vi "TDMS Cleanup EMG only.vi"(7 "Accel TDMS File":refnum<k34>, 8 "error in (no error)":errorcluster, 9 "Force TDMS File":refnum<k34>, 10 "TDMS File":path, 11 "Logging in":refnum<class "Logging.lvclass">) -> (0 "error out":errorcluster, 3 "Logging out":refnum<class "Logging.lvclass">)   [LabVIEW 2020, in "Logging.lvlib" / "Logging.lvclass"]
uses:
  Logging.lvclass
  C:/Program Files/National Instruments/LabVIEW 2020/vi.lib/ActorFramework/Actor/Actor.lvclass
  <vilib>/ActorFramework/Actor/Actor.lvclass/Actor.ctl
  <vilib>/ActorFramework/Message Enqueuer/Message Enqueuer.lvclass/Message Enqueuer.ctl
  Logging.lvclass/Logging.ctl
  <vilib>/ActorFramework/Message Enqueuer/Init from Existing Queue.vi
  <vilib>/ActorFramework/Message Enqueuer/Message Enqueuer.lvclass
  <vilib>/ActorFramework/Actor/Actor.lvclass
  Logging Messages/Convert to Excel Msg/Convert to Excel Msg.lvclass
panel:
  out "Numeric":i32
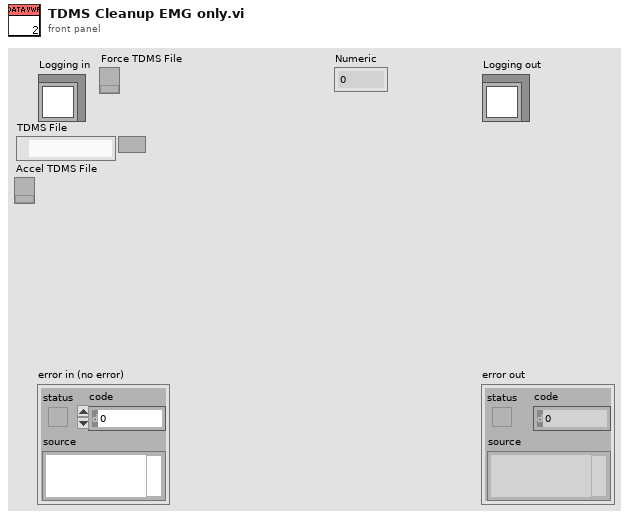
[diagram p1: front panel]
types:
  T1 = enum16{"open", "open or create", "create or replace", "create", "open (read-only)"}
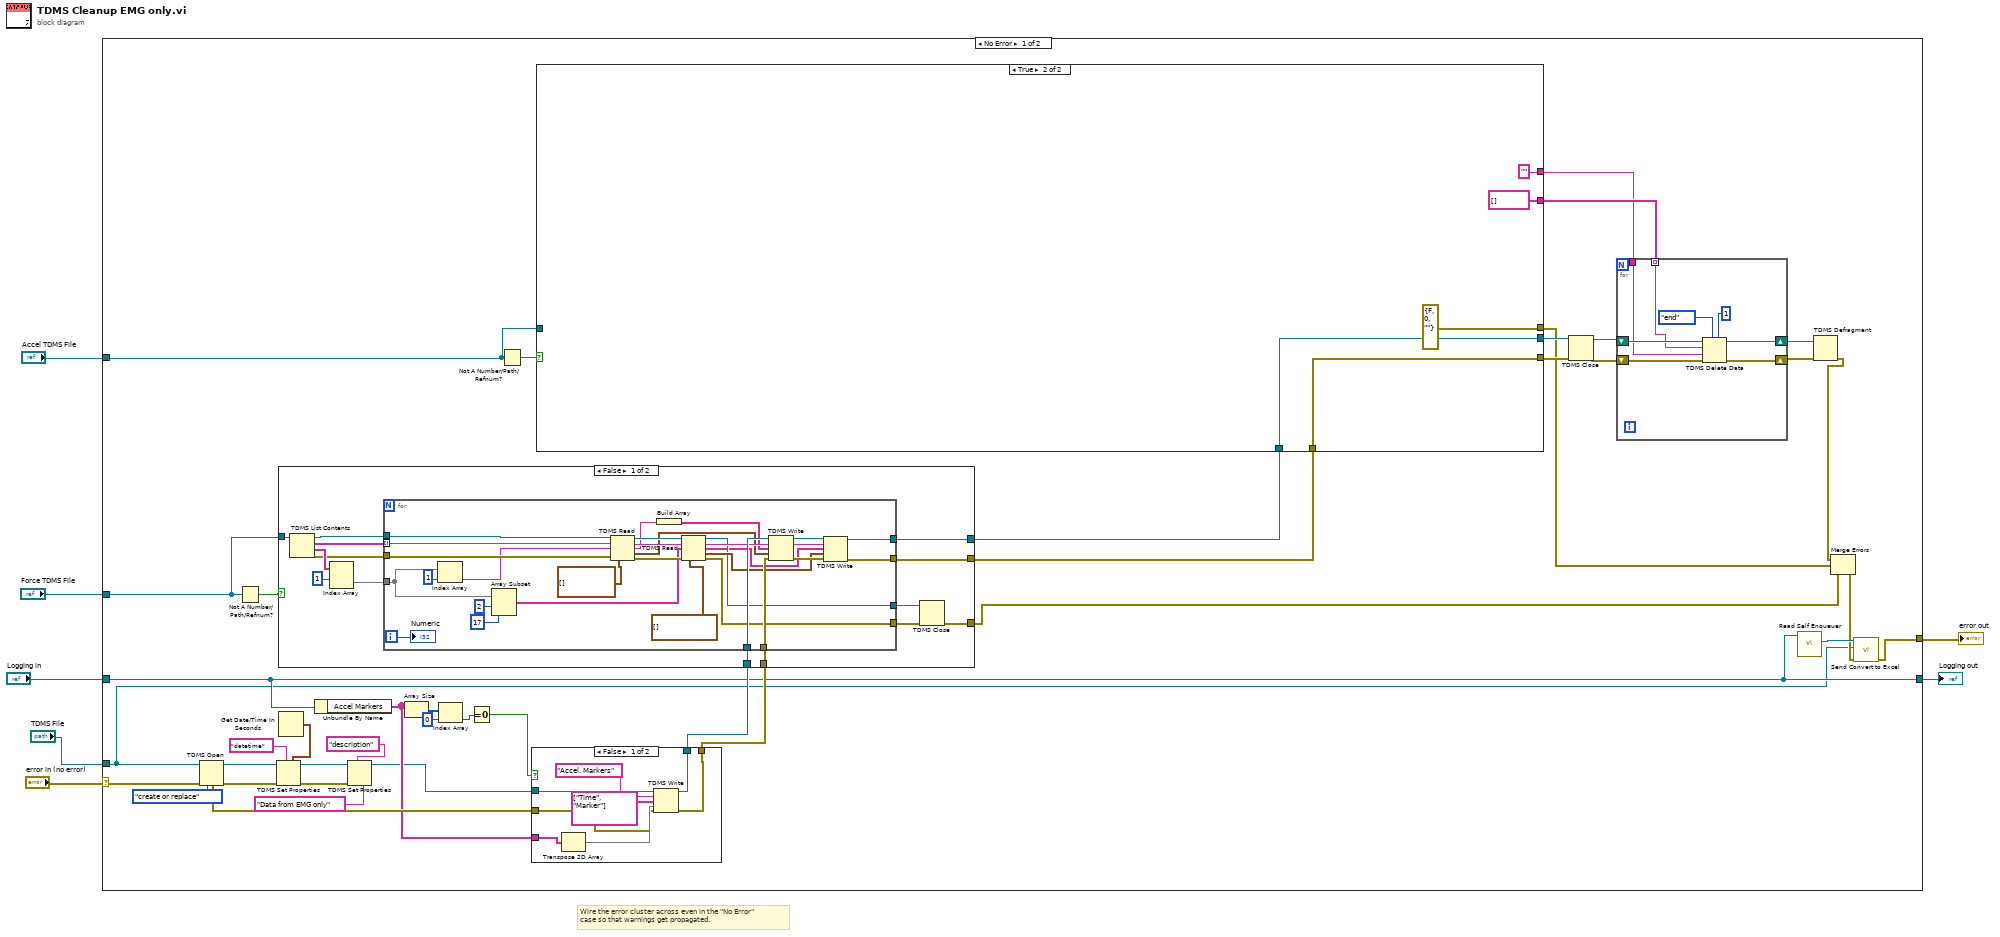
[diagram p0: block diagram]
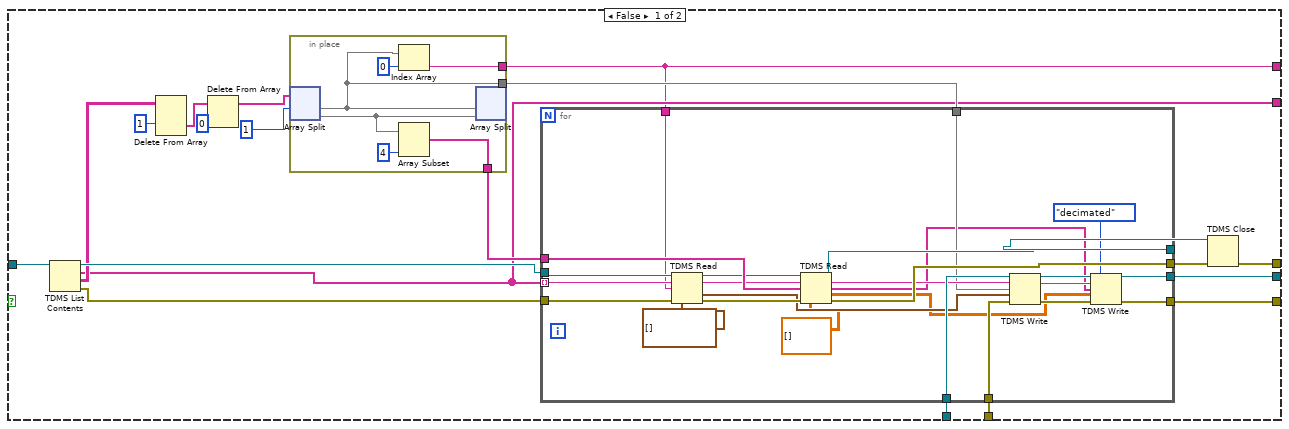
[diagram p2: hidden frame]
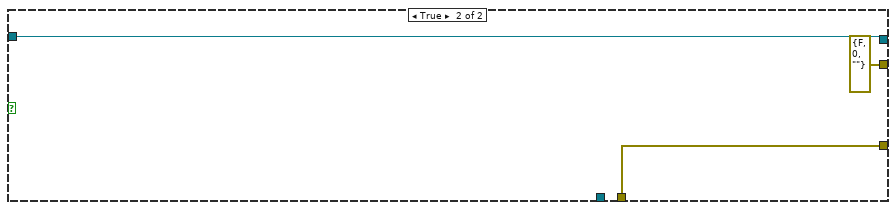
[diagram p3: hidden frame]
diagram:
  # "Wire the error cluster across even in the \"No Error\"\ncase so that warnings get propagated."
  n1 = case shown="No Error" "error in (no error)" {
    selector: "error in (no error)" -> [w41 w171]
    tunnel: [w15 w171] -> w6
    tunnel: [w18 w170] -> w4
    tunnel: "Logging in" -> [w18 w170]
    tunnel: "TDMS File" -> [w14 _]
    tunnel: "Force TDMS File" -> [w31 _]
    tunnel: "Accel TDMS File" -> [w21 _]
    frame No Error {
      n2 = TDMS Open(8:w41, 10:T1."create or replace" ("operation (0:open)"), 11:w14) -> (0:w46:errorcluster, 3:w47:refnum<k34>)  [unwired: 4 in]
      n3 = Not A Number/Path/Refnum?(number/path/refnum=w31) -> (NaN/Path/Refnum?=w32:bool)
      n4 = Get Date/Time In Seconds() -> (seconds since 1Jan1904=w44:timestamp)
      n5 = TDMS Set Properties(5:w44, 7:"datetime", 8:w46, 11:w47) -> (0:w42:errorcluster, 3:w43:refnum<k34>)  [unwired: 2 in, 2 out]
      n6 = Unbundle By Name(w18) -> ("Accel Markers"=w34:string[][])
      n7 = TDMS Set Properties(5:"Data from EMG only" ("property names"), 7:"description" ("property names"), 8:w42, 11:w43) -> (0:w35:errorcluster, 3:w33:refnum<k34>)  [unwired: 2 in, 2 out]
      n8 = Array Size(array=w34) -> (size(s)=w38:i32[])
      n9 = Index Array(array=w38, index=0) -> (element=w36:i32)
      n10 = Equal To 0?(x=w36) -> (x = 0?=w30:bool)
      n11 = Not A Number/Path/Refnum?(number/path/refnum=w21) -> (NaN/Path/Refnum?=w22:bool)
      n12 = case shown="False" w30 {
        tunnel: w33 -> [w167 w169]
        tunnel: w35 -> [w160 w168]
        tunnel: [w164 w169] -> w29
        tunnel: [w163 w168] -> w28
        tunnel: w34 -> [w162 _]
        frame False {
          n13 = Transpose 2D Array(2D array=w162) -> (transposed array=w161:string[][])
          n14 = TDMS Write(0:w167, 5:"Accel. Markers" ("group name in (Untitled)"), 7:string[] ["Time", "Marker"] ("channel name(s) in (Untitled)"), 9:w161, 11:w160) -> (4:w164:refnum<k34>, 15:w163:errorcluster)  [unwired: 1 in, 2 out]
        }
        frame True {
        }
      }
      n15 = case shown="False" w32 {
        tunnel: w31 -> [w126 w159]
        tunnel: w29 -> [w120 _]
        tunnel: w28 -> [w119 w157]
        tunnel: [w115 w157] -> w25
        tunnel: [w114 w159] -> w27
        tunnel: [w113 errorcluster {"status"=FALSE, "code"=0, "source"=""} ("error out")] -> w26
        frame False {
          n16 = TDMS List Contents(7:w126) -> (0:w121:errorcluster, 1:w124:string[][], 2:w123:string[], 3:w118:refnum<k34>)  [unwired: 2 in]
          n17 = Index Array(array=w124, index (row)=1) -> (element=w122:string[])  [unwired: 1 in]
          n18 = for {
            tunnel: w123 -> [w156] mode=indexing
            tunnel: w122 -> [w131]
            tunnel: w121 -> [w152]
            tunnel: w120 -> [w150]
            tunnel: w119 -> [w147]
            tunnel: w118 -> [w146]
            tunnel: [w138] -> w117
            tunnel: [w137] -> w116
            tunnel: [w136] -> w114
            tunnel: [w135] -> w113
            i -> [w133]
            n19 = Index Array(array=w131, index=1) -> (element=w130:string)
            n20 = Array Subset(array=w131, index=2, length=17) -> (w127:string[])
            n21 = TDMS Read(0:w146, 5:w156, 7:w130, 11:w152, 12:timestamp[] []) -> (4:w145:refnum<k34>, 6:w155:string, 8:w142:string, 10:w140:timestamp[], 15:w151:errorcluster)  [unwired: 3 in, 1 out]
            n22 = Build Array(w142) -> (w141:string[])
            n23 = TDMS Read(0:w145, 5:w155, 7:w127, 11:w151, 12:waveform(dbl)[] [] ("data")) -> (4:w138:refnum<k34>, 6:w144:string, 8:w132:string[], 10:w139:waveform(dbl)[], 15:w137:errorcluster)  [unwired: 3 in, 1 out]
            n24 = TDMS Write(0:w150, 5:w144, 7:w141, 9:w140, 11:w147) -> (4:w149:refnum<k34>, 6:w143:string, 15:w148:errorcluster)  [unwired: 1 in, 1 out]
            n25 = TDMS Write(0:w149, 5:w143, 7:w132, 9:w139, 11:w148) -> (4:w136:refnum<k34>, 15:w135:errorcluster)  [unwired: 1 in, 2 out]
            "Numeric" <- w133
          }
          n26 = TDMS Close(8:w116, 11:w117) -> (0:w115:errorcluster)  [unwired: 1 out]
        }
        frame True {
        }
      }
      n27 = case shown="True" w22 {
        tunnel: w21 -> [w76 _]
        tunnel: w27 -> [w74 w112]
        tunnel: [w73 w112] -> w24
        tunnel: w26 -> [w71 w111]
        tunnel: [w69 w111] -> w23
        tunnel: [w68 errorcluster {"status"=FALSE, "code"=0, "source"=""} ("error out")] -> w20
        tunnel: [w58 string[] [] ("group names")] -> w9
        tunnel: [w57 ""] -> w8
        frame False {
          n28 = TDMS List Contents(7:w76) -> (0:w59:errorcluster, 1:w64:string[][], 2:w58:string[], 3:w75:refnum<k34>)  [unwired: 2 in]
          n29 = Delete From Array(array=w64, index (row)=1) -> (deleted portion=w66:string[])  [unwired: 2 in, 1 out]
          n30 = Delete From Array(array=w66, index=0) -> (array with subset deleted=w63:string[])  [unwired: 1 in, 1 out]
          n31 = in-place {
            in-place-border: [w77] -> w61
            in-place-border: [w81] -> w57
            in-place-border: [w80] -> w60
            n32 = in-place-split #1(w63, 1) -> (w80:string[], w79:string[])
            n33 = Index Array(array=w80, index=0) -> (element=w81:string)
            n34 = Array Subset(array=w79, length=4) -> (w77:string[])  [unwired: 1 in]
            n35 = in-place-split #1(w80, w79) -> ()  [unwired: 2 out]
          }
          n36 = for {
            tunnel: w75 -> [w102]
            tunnel: w58 -> [w100] mode=indexing
            tunnel: w74 -> [w97]
            tunnel: [w107] -> w73
            tunnel: [w106] -> w72
            tunnel: w71 -> [w88]
            tunnel: [w105] -> w70
            tunnel: [w104] -> w69
            tunnel: w61 -> [w103]
            tunnel: w57 -> [w93]
            tunnel: w60 -> [w92]
            tunnel: w59 -> [w84]
            n37 = TDMS Read(0:w102, 5:w100, 7:w93, 11:w84, 12:timestamp[] []) -> (4:w101:refnum<k34>, 6:w99:string, 10:w87:timestamp[], 15:w98:errorcluster)  [unwired: 3 in, 2 out]
            n38 = TDMS Read(0:w101, 5:w99, 7:w103, 11:w98, 12:dbl[][] [] ("subarray")) -> (4:w106:refnum<k34>, 6:w95:string, 8:w90:string[], 10:w85:dbl[][], 15:w105:errorcluster)  [unwired: 3 in, 1 out]
            n39 = TDMS Write(0:w97, 5:w95, 7:w92, 9:w87, 11:w88) -> (4:w96:refnum<k34>, 6:w94:string, 15:w91:errorcluster)  [unwired: 1 in, 1 out]
            n40 = TDMS Write(0:w96, 1:enum16{"decimated", "interleaved"}."decimated" ("data layout (0:decimated)"), 5:w94, 7:w90, 9:w85, 11:w91) -> (4:w107:refnum<k34>, 15:w104:errorcluster)  [unwired: 2 out]
          }
          n41 = TDMS Close(8:w70, 11:w72) -> (0:w68:errorcluster)  [unwired: 1 out]
        }
        frame True {
        }
      }
      n42 = TDMS Close(8:w23, 11:w24) -> (0:w12:errorcluster, 3:w13:path)
      n43 = for {
        shift-right: [w53] -> w10
        shift-left: w12 -> [w56]
        shift-right: [w54] -> w11
        shift-left: w13 -> [w55]
        tunnel: w9 -> [w51] mode=indexing
        tunnel: w8 -> [w50]
        n44 = TDMS Delete Data(5:i64 1 ("count (-1: all)"), 7:enum16{"start", "end"}."end" ("from (0: start)"), 8:w56, 9:w50, 10:w51, 11:w55) -> (0:w53:errorcluster, 3:w54:path)  [unwired: 1 in]
      }
      n45 = call <vilib>:"Read Self Enqueuer.vi"("Actor"=w18) -> ("Self Enqueuer"=w17:refnum<class "Message Enqueuer.lvclass">)  [unwired: 10 in]
      n46 = TDMS Defragment(4:w10, 7:w11) -> (0:w19:errorcluster)
      n47 = Merge Errors(w19, w20, w25) -> (w16:errorcluster)
      n48 = call "Send Convert to Excel.vi"("error in (no error)"=w16, "Path to TDMS/TDM File"=w14, "Message Enqueuer in"=w17) -> ("error out"=w15:errorcluster)  [unwired: 7 in, 1 out]
    }
    frame Error {
    }
  }
  "error out" <- w6
  "Logging out" <- w4
